vi "更新信息.vi"(0 "MainPage 输入":refnum<class "MainPage.lvclass">, 1 "VISA串口名称":refnum<visa-resource-name>, 2 "服务端":T1, 3 "客服端":T2, 5 "error in (no error)":errorcluster caption="错误输入（无错误）", 10 "连接方式":enum16{"网口(客服端)", "网口(服务端)", "串口"}(ring)) -> (14 "MainPage 输出":refnum<class "MainPage.lvclass">, 19 "error out":errorcluster caption="错误输出")   [LabVIEW 2019, in "MainPage.lvlib" / "MainPage.lvclass"]
uses:
  MainPage.lvclass
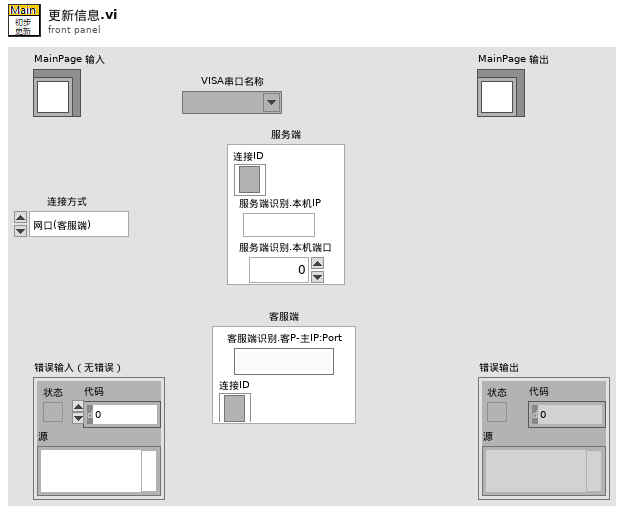
[diagram p1: front panel]
types:
  T1 = cluster{"连接ID":refnum<k5>, "服务端识别.本机IP":string, "服务端识别.本机端口":u16}
  T2 = cluster{"客服端识别.客P-主IP:Port":string, "连接ID":refnum<k5>}
  T3 = cluster{"串口正常？":bool, "寄存器模拟":u16[], "报文信息记录":string[][]}
  T4 = enum16{"ini", "读取", "写入-报文记录", "写入-寄存器模拟", "写入-串口状态", "增加报文记录"}
  T5 = enum16{"ini", "增加记录", "读取记录", "更改寄存器值", "更改接口状态", "更改报文信息", "增加报文信息"}
  T6 = cluster{"寄存器模拟":u16[], "串口正常？":bool, "报文信息记录":string[][]}
  T7 = cluster{"本机IP":string, "本机端口":u16, "当前目标":string}
  T8 = typedef "MainPage.lvlib/MainPage.lvclass/DataRef_通讯接口.ctl" = cluster{"连接方式":enum16{"串口", "网口(客服端)", "网口(服务端)"}, "VISA串口名称":refnum<visa-resource-name>, "服务端识别":cluster{"本机IP":string, "本机端口":u16, "当前目标":string}, "客服端识别":cluster{"客P-主IP:Port":string}, "服务端记录":cluster{"服务端侦听ID":refnum<k5>, "服务端接口记录":map{string, refnum<k5>}}, "客服端记录":map{string, refnum<k5>}}
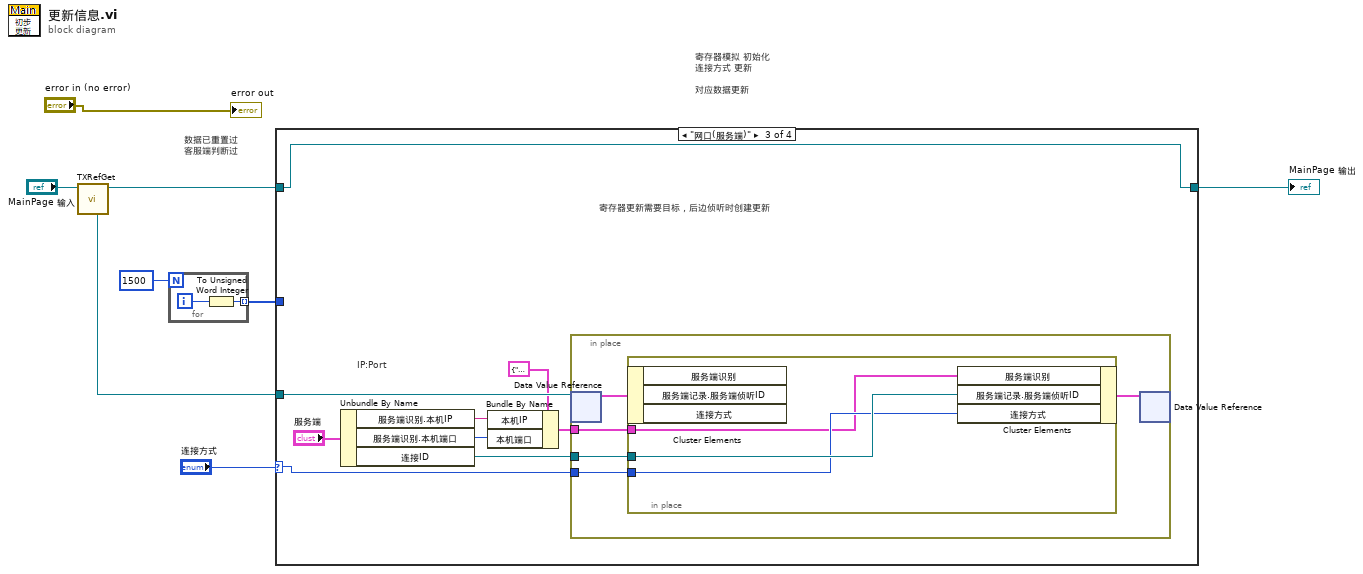
[diagram p0: block diagram]
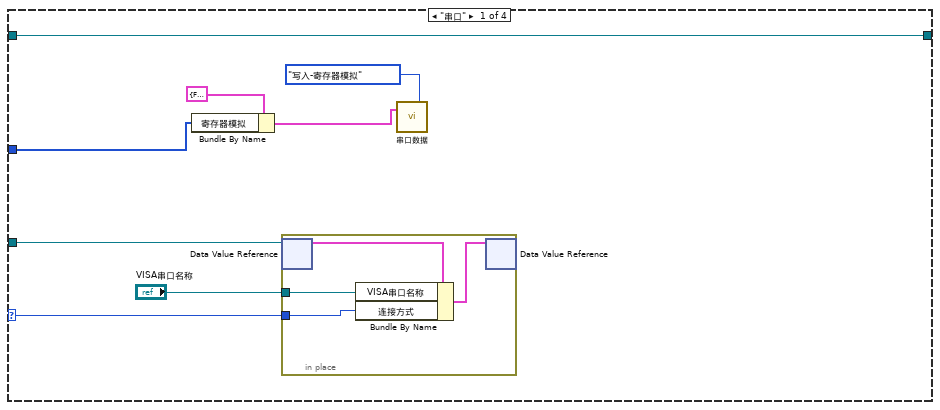
[diagram p2: hidden frame]
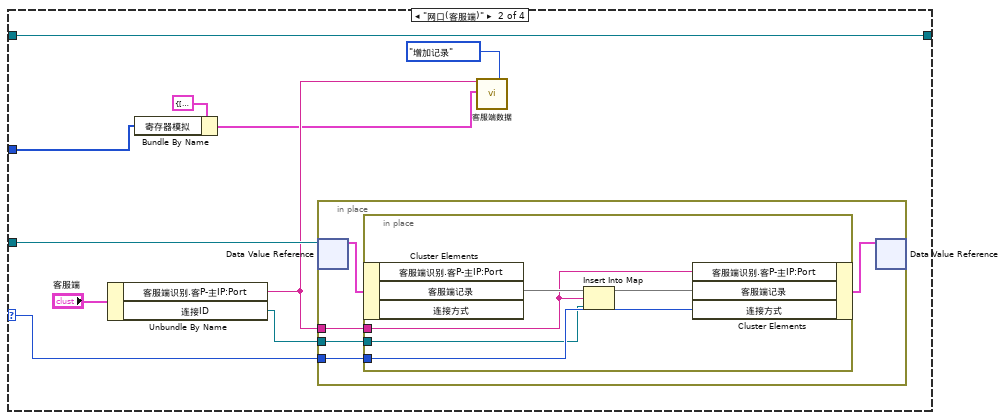
[diagram p3: hidden frame]
diagram:
  # "寄存器模拟 初始化\n连接方式 更新\n\n对应数据更新"
  # "数据已重置过\n客服端判断过"
  n1 = call-dynamic "TXRefGet.vi"("MainPage 输入"="MainPage 输入") -> ("MainPage 输出"=w1:refnum<class "MainPage.lvclass">, "引用"=w5:refnum<data-value>)  [unwired: 6 in, 3 out]
  n2 = for {
    N: 1500 -> [_]
    tunnel: [w9] -> w2 mode=indexing
    i -> [w10]
    n3 = To Unsigned Word Integer(number=w10) -> (unsigned 16bit integer=w9:u16)
  }
  n4 = case shown="\"网口(服务端)\"" "连接方式" {
    selector: "连接方式" -> [w15 w30 w48 _]
    tunnel: [w18 w32 w43 w60] -> w8
    tunnel: w1 -> [w18 w32 w43 w60]
    tunnel: w5 -> [w17 w31 w51 _]
    tunnel: w2 -> [w12 w24 _ _]
    frame "串口" {
      n5 = Bundle By Name(cluster=T3 {"串口正常？"=FALSE, "寄存器模拟"=[], "报文信息记录"=[]} ("串口输入"), "寄存器模拟"=w12) -> (w11:T3)
      n6 = in-place {
        in-place-border: "VISA串口名称" -> [w20]
        in-place-border: w15 -> [w19]
        n7 = in-place-dvr #1(w17) -> (w21:T8)  [unwired: 1 out]
        n8 = Bundle By Name(cluster=w21, "VISA串口名称"=w20, "连接方式"=w19) -> (w22:T8)
        n9 = in-place-dvr #1(w22) -> ()  [unwired: 2 out]
      }
      n10 = call "串口数据.vi"("串口输入"=w11, "枚举"=T4."写入-寄存器模拟") -> ()  [unwired: 17 in, 1 out]
    }
    frame "网口(客服端)" {
      n11 = Unbundle By Name("客服端") -> ("客服端识别.客P-主IP:Port"=w25:string, "连接ID"=w28:refnum<k5>)
      n12 = Bundle By Name(cluster=T6 {"寄存器模拟"=[], "串口正常？"=FALSE, "报文信息记录"=[]} ("值"), "寄存器模拟"=w24) -> (w23:T6)
      n13 = in-place {
        in-place-border: w30 -> [w35]
        in-place-border: w28 -> [w34]
        in-place-border: w25 -> [w33]
        n14 = in-place-dvr #2(w31) -> (w37:T8)  [unwired: 1 out]
        n15 = in-place {
          in-place-border: w35 -> [w40]
          in-place-border: w34 -> [w39]
          in-place-border: w33 -> [w38]
          n16 = in-place-cluster #3(w37) -> ("客服端记录"=w42:map{string, refnum<k5>})  [unwired: 2 out]
          n17 = Insert Into Map(map in=w42, key=w38, value=w39) -> (map out=w41:map{string, refnum<k5>})  [unwired: 2 out]
          n18 = in-place-cluster #3("客服端识别.客P-主IP:Port"=w38, "客服端记录"=w41, "连接方式"=w40) -> (w36:T8)
        }
        n19 = in-place-dvr #2(w36) -> ()  [unwired: 2 out]
      }
      n20 = call "客服端数据.vi"("客P-主IP:P"=w25, "数据输入"=w23, "枚举"=T5."增加记录") -> ()  [unwired: 15 in, 2 out]
    }
    frame "网口(服务端)" {
      # "寄存器更新需要目标，后边侦听时创建更新"
      # "IP:Port"
      n21 = Unbundle By Name("服务端") -> ("服务端识别.本机IP"=w46:string, "服务端识别.本机端口"=w45:u16, "连接ID"=w49:refnum<k5>)
      n22 = Bundle By Name(cluster=T7 {"本机IP"="", "本机端口"=0, "当前目标"=""} ("服务端识别"), "本机IP"=w46, "本机端口"=w45) -> (w44:T7)
      n23 = in-place {
        in-place-border: w49 -> [w54]
        in-place-border: w48 -> [w53]
        in-place-border: w44 -> [w52]
        n24 = in-place-dvr #4(w51) -> (w56:T8)  [unwired: 1 out]
        n25 = in-place {
          in-place-border: w54 -> [w59]
          in-place-border: w53 -> [w58]
          in-place-border: w52 -> [w57]
          n26 = in-place-cluster #5(w56) -> ()  [unwired: 3 out]
          n27 = in-place-cluster #5("服务端识别"=w57, "服务端记录.服务端侦听ID"=w59, "连接方式"=w58) -> (w55:T8)
        }
        n28 = in-place-dvr #4(w55) -> ()  [unwired: 2 out]
      }
    }
    frame Default {
    }
  }
  "MainPage 输出" <- w8
  "error out" <- "error in (no error)"
